vi "Analyze Data.vi"(8 "error in":errorcluster, 11 "CRDS in":refnum<class "CRDS.lvclass">) -> (0 "error out":errorcluster, 3 "CRDS out":refnum<class "CRDS.lvclass">)   [LabVIEW 2014, in "CRDS Lib.lvlib" / "CRDS.lvclass"]
doc: "Analyze Data takes the stored ringdown data (1000 shots per cell) and:\n1) Calculates the ringdown decay constant tau\n2) Averages tau0 data as necessary\n3) Corrects the tau data for Rayleigh scattering\n4) Stores a 1-D array of taus returned on a 1 kHz basis (8k taus) if a jump drive (U:) is connected\n5) Flattens the data into a string and stuffs the string into the <b>data</b> shared variable for display on the UI.\n\nThis VI will not be called if the data is not \"good\" (that is, if an error was thrown in the <B>Get Data</B> routine. If an error is thrown while the data is being retrieved, then the data will not be sent to the UI."
uses:
  CRDS.lvclass
  Instrument/Instrument.lvclass/Instrument.ctl
  Data/Main/CRDS Data.lvclass
  Cell/CRDS Cell.lvclass/CRDS Cell.ctl
  Instrument/Write Data.vi
  Read Cells.vi
  Data/Main/Read filter.vi
  Write Cells.vi
  Cell/CRDS Cell.lvclass
  Data/Data.lvclass
  Instrument/Instrument.lvclass
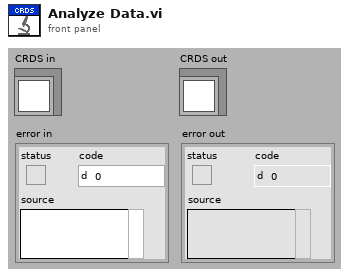
[diagram p1: front panel]
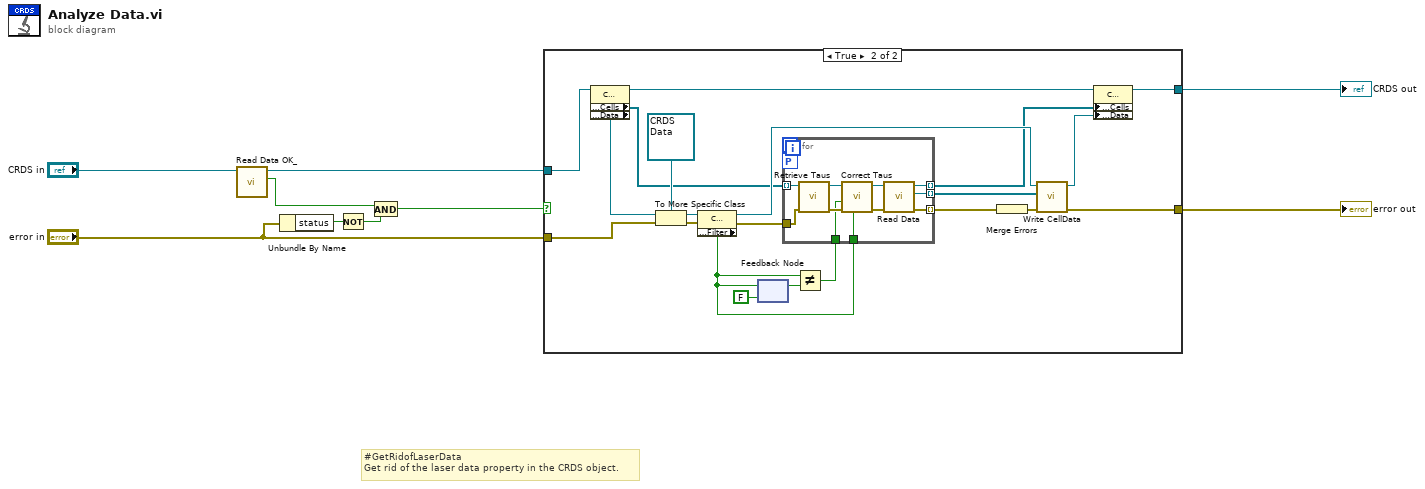
[diagram p0: block diagram]
diagram:
  # "#GetRidofLaserData\nGet rid of the laser data property in the CRDS object."
  n1 = call "Read Data OK_.vi"("Instrument in"="CRDS in") -> ("Data OK?"=w1:bool, "Instrument out"=w2:refnum<class "CRDS.lvclass">)  [unwired: 8 in, 1 out]
  n2 = Unbundle By Name("error in") -> ("status"=w5:bool)
  n3 = Not(x=w5) -> (.not. x?=w4:bool)
  n4 = And(x=w1, y=w4) -> (x .and. y?=w3:bool)
  n5 = case shown="True" w3 {
    tunnel: w2 -> [w11 w31]
    tunnel: "error in" -> [w10 w14]
    tunnel: [w11 w29] -> w8
    tunnel: [w10 w32] -> w7
    frame False {
    }
    frame True {
      n6 = property class="CRDS"(reference=w31) -> (reference out=w15:refnum<class "CRDS.lvclass">, "Data Access:Cells"=w12:refnum<class "CRDS Cell.lvclass">[], "Accessors:Data"=w19:refnum<class "Data.lvclass">)  [unwired: 1 in, 1 out]
      n7 = To More Specific Class(target class=refnum<class "CRDS Data.lvclass"> refnum ("reference out"), reference=w19, error in=w14) -> (specific class reference=w18:refnum<class "CRDS Data.lvclass">, error out=w13:errorcluster)
      n8 = property class="CRDS"(reference=w18, error in=w13) -> (reference out=w20:refnum<class "CRDS Data.lvclass">, error out=w22:errorcluster, "Accessors:Filter"=w23:bool)
      n9 = feedback #1(FALSE ("filter")) -> (w26:bool)
      n10 = feedback-in #1(w23) -> ()
      n11 = Not Equal?(x=w23, y=w26) -> (x != y?=w24:bool)
      n12 = for "Initial extinction calculation" {
        tunnel: w12 -> [w40] mode=indexing
        tunnel: w22 -> [w33]
        tunnel: w23 -> [w43]
        tunnel: [w37] -> w17 mode=indexing
        tunnel: [w36] -> w28 mode=indexing
        tunnel: [w35] -> w27 mode=indexing
        tunnel: w24 -> [w34]
        workers-P: _ -> [_]
        n13 = call "Retrieve Taus.vi"("error in"=w33, "CRDS Cell in"=w40) -> ("error out"=w41:errorcluster, "CRDS Cell out"=w42:refnum<class "CRDS Cell.lvclass">)  [unwired: 7 in, 1 out]
        n14 = call "Correct Taus.vi"("Filter?"=w43, "error in"=w41, "filter changed?"=w34, "CRDS Cell in"=w42) -> ("error out"=w38:errorcluster, "CRDS Cell out"=w39:refnum<class "CRDS Cell.lvclass">)  [unwired: 6 in]
        n15 = call "Read Data.vi"("error in"=w38, "CRDS Cell in"=w39) -> ("error out"=w36:errorcluster, "CRDS Cell"=w35:refnum<class "CRDS Cell Data.lvclass">, "CRDS Cell out"=w37:refnum<class "CRDS Cell.lvclass">)  [unwired: 7 in]
      }
      n16 = Merge Errors(w28) -> (w21:errorcluster)
      n17 = call "Write CellData.vi"("error in"=w21, "CellData"=w27, "CRDS Data in"=w20) -> ("error out"=w32:errorcluster, "CRDS Data out"=w16:refnum<class "CRDS Data.lvclass">)  [unwired: 7 in]
      n18 = property class="CRDS"(reference=w15, "Data Access:Cells"=w17, "Accessors:Data"=w16) -> (reference out=w29:refnum<class "CRDS.lvclass">)  [unwired: 1 in, 1 out]
    }
  }
  "error out" <- w7
  "CRDS out" <- w8
